vi "MergeFileAutoConfig.vi"(4 "error in (no error)":errorcluster, 6 "test num":u32, 7 "ProjetIN":string) -> (0 "error out":errorcluster, 2 "MergeFileConfigOUT":T1, 3 "ProjetOUT":string)   [LabVIEW 2017]
uses:
  DefDeType/MergeFileConfig.ctl
  DefDeType/WhichPath.ctl
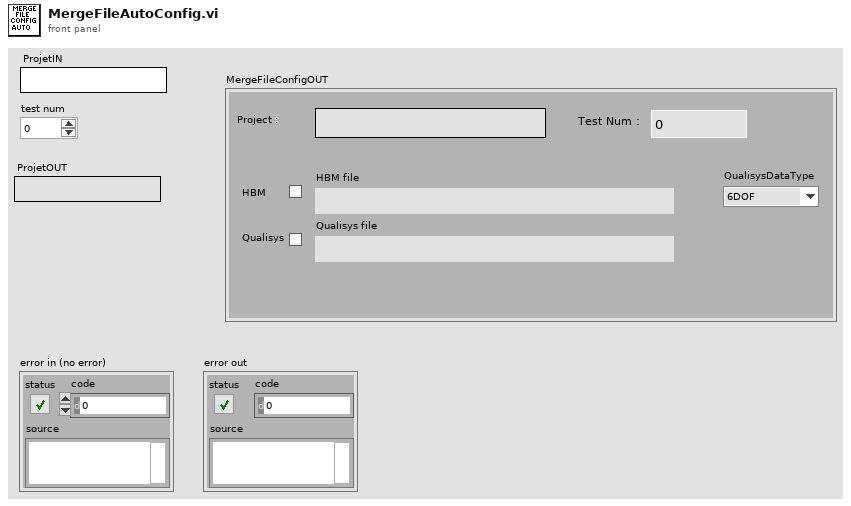
[diagram p1: front panel]
types:
  T1 = typedef "MergeFileConfig.ctl" = cluster{"Test Num : ":u32, "Project :":string, "Qualisys file":path, "HBM file":path, "QualisysDataType":enum16{"6DOF", "3DTracking", "6DOF + 3D"}, "Qualisys":bool, "HBM":bool}
  T2 = typedef "WhichPath.ctl" = enum16{"DossierProjet", "Config", "Meas", "MeasPCI", "MeasCRIO1", "MeasCRIO2", "MeasQualisys", "MeasHBM", "MeasTDMS", "Fig", "Res"}
  T3 = typedef "ConfigTotale.ctl" = cluster{"VoltageChannels":T4, "WheastoneBridgeChannels":T5, "Configuration":T6}
  T4 = typedef "VoltageChannels.ctl" = cluster{"ChannelNames":string[], "Sensitivity(Unit/V)":dbl[], "AutoZero":bool[], "ChannelUnits":string[], "Offsets(Units)":dbl[], "Graph Num":u8[]}
  T5 = typedef "WBridgeChannels.ctl" = cluster{"ChannelNames":string[], "Sensitivity(Unit/V)":dbl[], "AutoZero":bool[], "ChannelUnits":string[], "Offsets(Units)":dbl[], "Graph Num":u8[]}
  T6 = typedef "Configuration.ctl" = cluster{"AcqSamplingRate(Hz)":u32, "AcqTime(s)":u32, "Trigger":bool, "NbVoltageChannels":u32, "NbWBridgeChannels":u32, "Qualisys":bool, "Hexapode":bool, "FinalSamplingRate(Hz)":u32, "QualisysDataType":enum16{"6DOF", "3DTracking", "6DOF + 3D"}, "Nortek":bool, "HBM":bool}
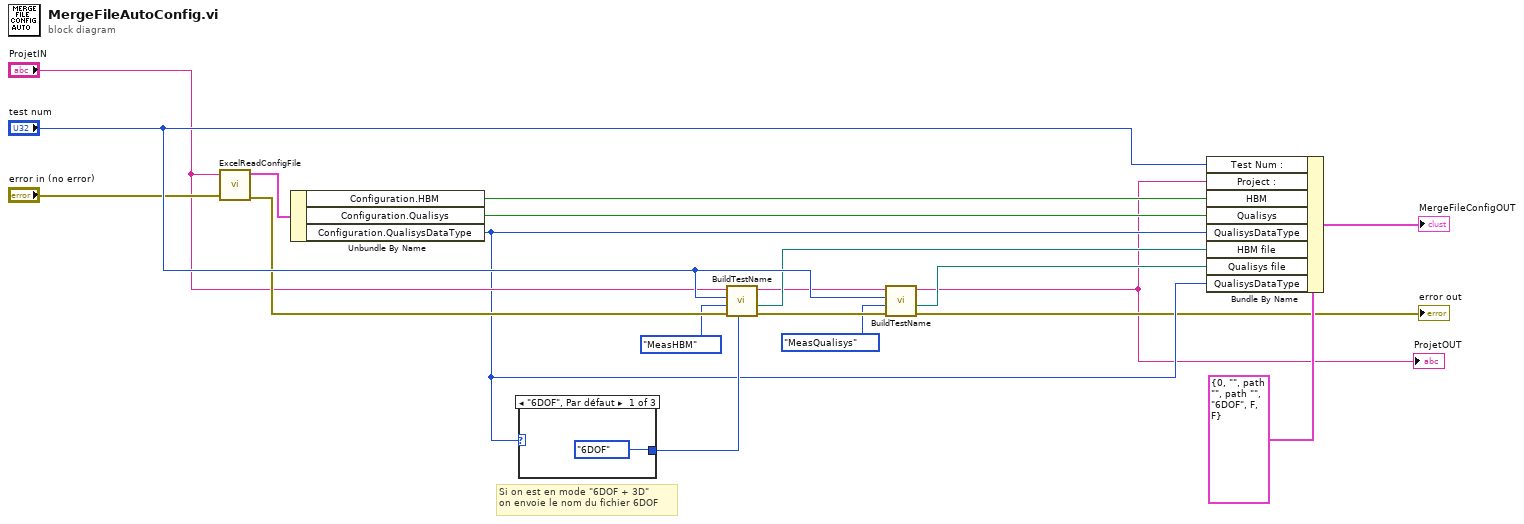
[diagram p0: block diagram]
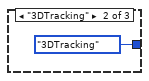
[diagram p2: hidden frame]
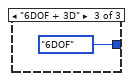
[diagram p3: hidden frame]
diagram:
  # "Si on est en mode \"6DOF + 3D\" \non envoie le nom du fichier 6DOF"
  n1 = call "ExcelReadConfigFile.vi"("NomProjet"="ProjetIN", "error in (no error)"="error in (no error)") -> ("ConfigurationTotale"=w8:T3, "error out"=w17:errorcluster)  [unwired: 3 in]
  n2 = Unbundle By Name(w8) -> ("Configuration.HBM"=w9:bool, "Configuration.Qualisys"=w10:bool, "Configuration.QualisysDataType"=w4:enum16{"6DOF", "3DTracking", "6DOF + 3D"})
  n3 = case shown="\"6DOF\", Par défaut" w4 {
    tunnel: [enum16{"6DOF", "3DTracking"}."6DOF" ("QualisysDataType") enum16{"6DOF", "3DTracking"}."3DTracking" ("QualisysDataType") enum16{"6DOF", "3DTracking"}."6DOF" ("QualisysDataType")] -> w5
    frame "6DOF", Default {
    }
    frame "3DTracking" {
    }
    frame "6DOF + 3D" {
    }
  }
  n4 = call "BuildTestName.vi"("QualisysDataType"=w5, "entrée d'erreur"=w17, "WhichPath?"=WhichPath."MeasHBM", "NextTestNum"="test num", "NomProjet"="ProjetIN") -> ("sortie d'erreur"=w13:errorcluster, "cheminProchainFichier"=w15:path, "NomProjetOut"=w14:string)  [unwired: 1 out]
  n5 = call "BuildTestName.vi"("entrée d'erreur"=w13, "WhichPath?"=WhichPath."MeasQualisys", "NextTestNum"="test num", "NomProjet"=w14) -> ("sortie d'erreur"=→"error out":errorcluster, "cheminProchainFichier"=w16:path, "NomProjetOut"=w1:string)  [unwired: 1 in, 1 out]
  "ProjetOUT" <- w1
  n6 = Bundle By Name(cluster=T1 {"Test Num : "=0, "Project :"="", "Qualisys file"=path "", "HBM file"=path "", "QualisysDataType"=enum."6DOF", "Qualisys"=FALSE, "HBM"=FALSE} ("MergeFileConfig 2"), "Test Num :"="test num", "Project :"=w1, "HBM"=w9, "Qualisys"=w10, "QualisysDataType"=w4, "HBM file"=w15, "Qualisys file"=w16, "QualisysDataType"=w4) -> (→"MergeFileConfigOUT":T1)
